vi "ciacs_forward_and_back_calc.vi"() -> ()   [LabVIEW 2011]
uses:
  cm2nm_sample_set.ctl
  cm2nm_coordinate_information_v2.ctl
  Instrument_type_enum_v2.ctl
  <vilib>/Utility/xml.llb/Read From XML File(string).vi
panel:
  out "Sample Information":T1={"Sample Name/ID"="Diffusion_sample", "Notes on Sample"="", "Session_list"=[{"Instrument"=2, "Session_data_base"=path "/INL Macintosh/Users/timothymcjunkin/Desktop/Diffusion couple/JEOL 7000F SEM 9-3-10/Jeol_9-3-10.xml", "Session Name/ID"="Initial Joel location"}, {"Instrument"=3, "Session_data_base"=path "/INL Macintosh/Users/timothymcjunkin/Desktop/Diffusion couple/MXRD 9-13-10/xrd_session.xlm", "Session Name/ID"="xrd_test"}, {"Instrument"=2, "Session_data_base"=path "/INL Macintosh/Users/timothymcjunkin/Desktop/Diffusion couple/JEOL 7000F SEM 9-3-10/Corrected_9-3-10.xlm", "Session Name/ID"="Correct_Abs_position"}]} {"Session_list"."Instrument" items=["Unknown", "Phillips SEM IRC", "JEOL 7000F EML_MFC", "MXRD MFC", "JEOL_EPMA"]}
  out "error out 3":errorcluster
  in  "Sample_data_base":path=path "/INL Macintosh/Users/timothymcjunkin/Desktop/diff_couple"
  in  "Array":T2[](array[typedef])
  in  "Sample_Information":T1={"Sample Name/ID"="Granite 5 compare sessions 4 and 5", "Notes on Sample"="Sample was physically rotated relative to the coordinate system between sessions 4 and 5.", "Session_list"=[{"Instrument"=0, "Session_data_base"=path "/Documents and Settings/jannde/Desktop/Karens granite session 4 session5/Session 4/Session 4.xml", "Session Name/ID"="Session 4"}, {"Instrument"=0, "Session_data_base"=path "/Documents and Settings/jannde/Desktop/Karens granite session 4 session5/Session 5/Session 5.xml", "Session Name/ID"="Session 5"}, {"Instrument"=0, "Session_data_base"=path "/Documents and Settings/jannde/Desktop/Karens granite session 4 session5/Session 6/Session 6.xml", "Session Name/ID"="Session 6"}]}
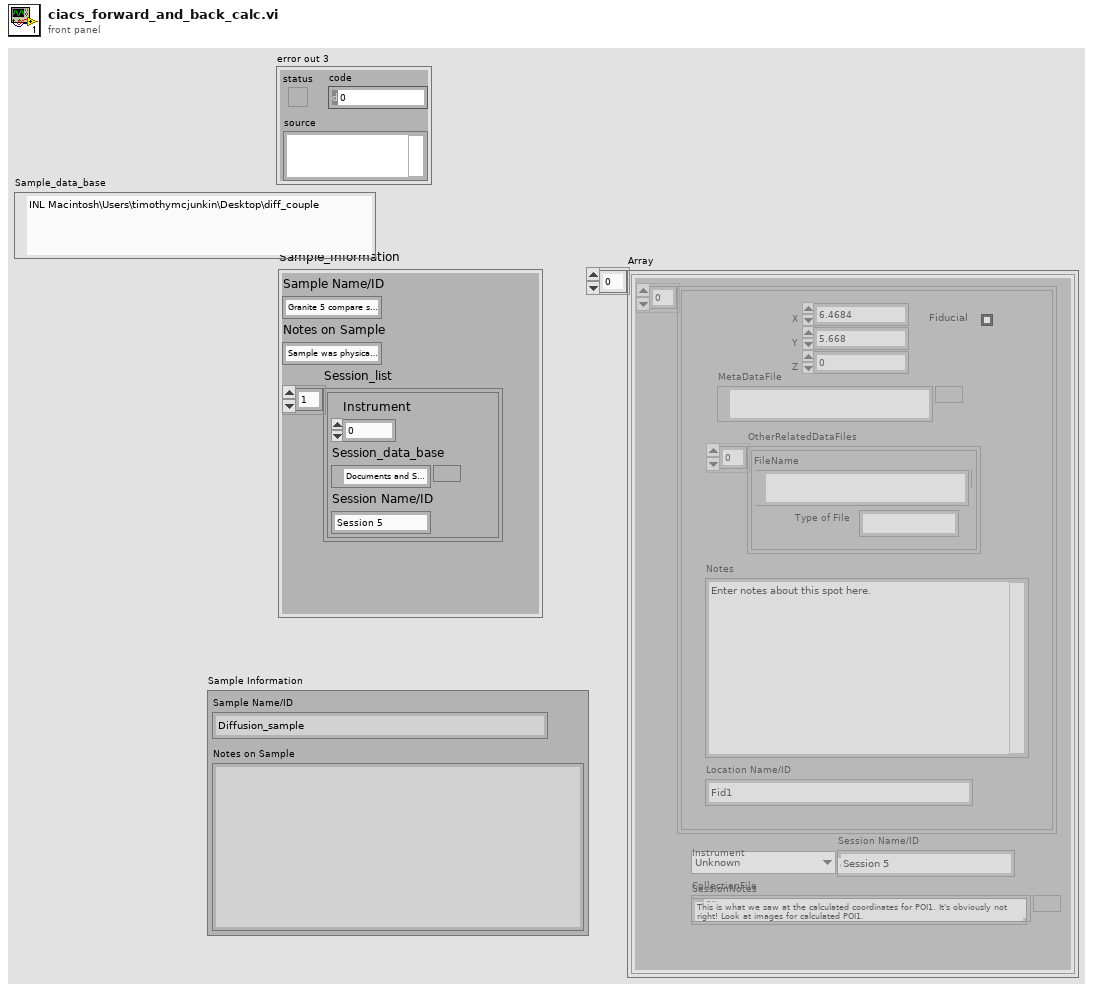
[diagram p1: front panel]
types:
  T1 = cluster{"Sample Name/ID":string, "Notes on Sample":string, "Session_list":cluster{"Instrument":u16, "Session_data_base":path, "Session Name/ID":string}[]}
  T2 = typedef "cm2nm_sample_set.ctl" = cluster{"CollectionOfPoints":T3[], "Instrument":T4, "CollectionFile":path, "Session Name/ID":string, "SessionNotes":string}
  T3 = typedef "cm2nm_coordinate_information_v2.ctl" = cluster{"MetaDataFile":path, "X":dbl, "Y":dbl, "Z":dbl, "Group":i32, "Rotation":dbl[unit], "Fiducial":bool, "Magnification":dbl, "Working_Distance":dbl, "Notes":string, "Location Name/ID":string, "OtherRelatedDataFiles":cluster{"Type of File":string, "FileName":path}[], "Available":bool}
  T4 = typedef "Instrument_type_enum_v2.ctl" = enum16{"Unknown", "Philips FEI SEM IRC", "JEOL 7000F EML_MFC", "MXRD MFC", "JEOL_EPMA"}
  T5 = cluster{"Instrument":u16, "Session_data_base":path, "Session Name/ID":string}[]
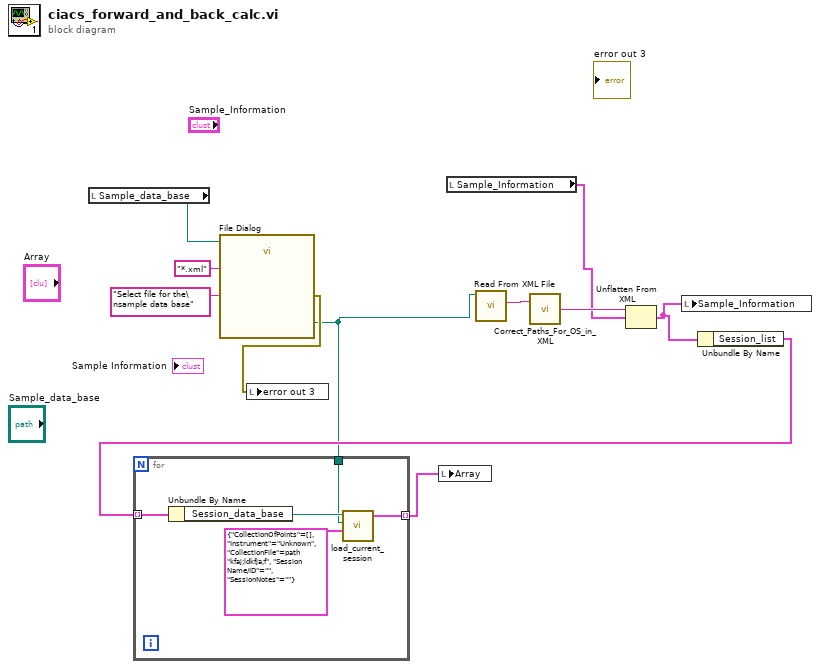
[diagram p0: block diagram]
diagram:
  n1 = local read "Sample_data_base"() -> (w11:path)
  n2 = call "File Dialog"("start path"=w11, "prompt"="Select file for the\nsample data base", "pattern (all files)"="*.xml") -> ("selected path"=w3:path, "error out"=w8:errorcluster)  [unwired: 9 in, 2 out]
  n3 = local write "error out 3"(w8) -> ()
  n4 = local read "Sample_Information"() -> (w1:T1)
  n5 = call-poly <vilib>:"Read From XML File.vi"("XML File Path"=w3) -> ("XML Elements"=w6:string)  [unwired: 1 in, 9 out]
  n6 = call "Correct_Paths_For_OS_in_XML.vi"("XML Elements"=w6) -> ("String"=w7:string)  [unwired: 1 in]
  n7 = Unflatten From XML(xml string=w7, type=w1) -> (value=w5:T1)  [unwired: 1 in, 1 out]
  n8 = local write "Sample_Information"(w5) -> ()
  n9 = Unbundle By Name(w5) -> ("Session_list"=w4:T5)
  n10 = for {
    tunnel: w4 -> [w16] mode=indexing
    tunnel: w3 -> [w14]
    tunnel: [w12] -> w2 mode=indexing
    n11 = Unbundle By Name(w16) -> ("Session_data_base"=w15:path)
    n12 = call "load_current_session.vi"("Current Session Information"=T2 {"CollectionOfPoints"=[], "Instrument"=enum."Unknown", "CollectionFile"=path "kfaj;ldkfja;f", "Session Name/ID"="", "SessionNotes"=""}, "TopLevelDataFilePath"=w14, "just a file"=w15) -> ("Sample Set"=w12:T2)  [unwired: 1 in, 2 out]
  }
  n13 = local write "Array"(w2) -> ()
